vi "RSNRPZ Get Test Deviation.vi"(8 "error in (no error)":errorcluster, 9 "Channel (1)":i32=1, 11 "VISA session":refnum<visa-resource-name> caption="VISA resource name") -> (0 "error out":errorcluster, 2 "Test Deviation":dbl format="%^.3e", 3 "dup VISA session":refnum<visa-resource-name> caption="VISA resource name")   [LabVIEW 2010]
doc: "This VI first does an internal heater test with CAL:TEST and returns the relative deviation between the test result and the result that was measured in the calibration lab during sensor calibration.\n\nNote:\n\n1) This VI is available only for NRP-Z56 and NRP-Z57.\n\nRemote-control command(s):\nCAL:TEST:DEV?"
uses:
  rsnrpz_32.dll
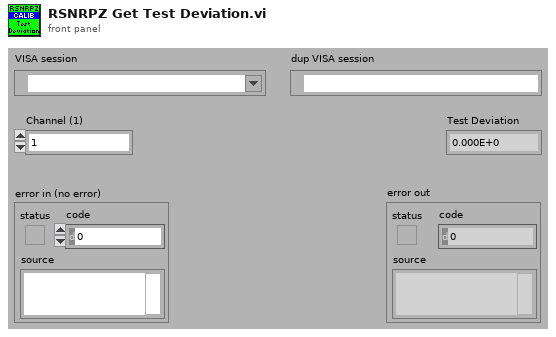
[diagram p1: front panel]
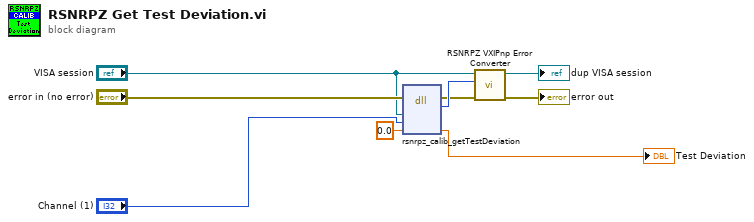
[diagram p0: block diagram]
diagram:
  n1 = dll-call lib="rsnrpz_32.dll" fn="rsnrpz_calib_getTestDeviation"(error in="error in (no error)", "Instrument Handle"="VISA session", "Channel"="Channel (1)", "Test Deviation"=0.0) -> (error out=w5:errorcluster, w7:i32, "Test Deviation"=→"Test Deviation":dbl)  [unwired: 4 in, 1 out]
  n2 = call <instrlib>:"RSNRPZ VXIPnp Error Converter.vi"("error in"=w5, "VXIPnp error code"=w7, "VISA session"="VISA session") -> ("error out"=→"error out":errorcluster, "dup VISA session"=→"dup VISA session":refnum<visa-resource-name>)  [unwired: 7 in]
